vi "OAT Linear Avg Level.vi"(0 "scaled signal [EU]":dbl[](array[numeric]) format="%.2f", 1 "time constant [ms]":dbl=125.0 min=0.0 format="%.2f", 2 "sampling frequency [Hz]":dbl=10000.0 format="%.2f", 4 "init/cont (init:F)":bool) -> (6 "linear avg level [EU^2 rms]":dbl[](array[numeric]) format="%.2f", 7 "actual time constant [ms]":dbl=125.0 format="%.2f")   [LabVIEW 2017, in "SoundVib_Gabor.lvlib"]
doc: "This VI computes the exponential averaged level of the input signal X, based on the selected exponential averaging mode, and returns this level for the entire signal..\n\nThe initial filter state and final filter state keep track of the internal state of the filter to insure continuous operation of the filter (if continuous mode is used)."
uses:
  <vilib>/addons/Sound and Vibration/Order Analysis/Gabor Order Tracking/SoundVib_Gabor.lvlib
  <vilib>/Analysis/3filter.llb/IIR Filter (DBL).vi
  <vilib>/Analysis/NI_AALBase.lvlib
panel:
  in  "exponential mode":enum16{"Slow", "Fast", "Impulse", "Custom"}(ring)=enum."Custom"
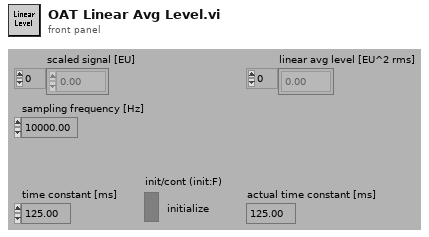
[diagram p1: front panel]
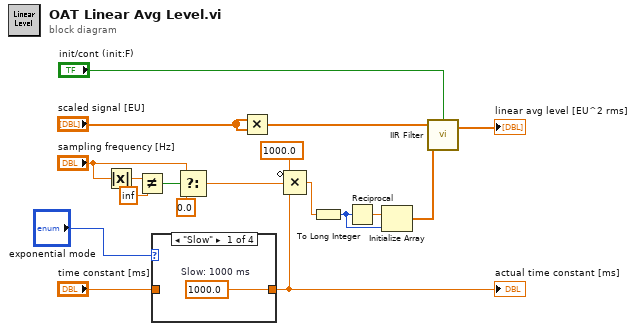
[diagram p0: block diagram]
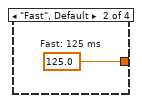
[diagram p2: hidden frame]
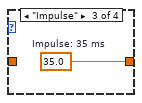
[diagram p3: hidden frame]
diagram:
  n1 = Absolute Value(x="sampling frequency [Hz]") -> (abs(x)=w6:dbl)
  n2 = Not Equal?(x=w6, y=inf) -> (x != y?=w4:bool)
  n3 = case shown="\"Slow\"" "exponential mode" {
    tunnel: [w19 w20 w21 w22] -> w12
    tunnel: "time constant [ms]" -> [_ _ _ w22]
    frame "Slow" {
      w19 = 1000.0  # Slow: 1000 ms
    }
    frame "Fast", Default {
      w20 = 125.0  # Fast: 125 ms
    }
    frame "Impulse" {
      w21 = 35.0  # Impulse: 35 ms
    }
    frame "Custom" {
    }
  }
  "actual time constant [ms]" <- w12
  n4 = Select(t="sampling frequency [Hz]", s=w4, f=0.0) -> (s? t:f=w1:dbl)
  n5 = Multiply(x="scaled signal [EU]", y="scaled signal [EU]") -> (x*y=w9:dbl[])
  n6 = Compound Arithmetic op=MULTIPLY(invert 1000.0 ("Input"), w1, w12) -> (w15:dbl)
  n7 = To Long Integer(number=w15) -> (32bit integer=w13:i32)
  n8 = Reciprocal(x=w13) -> (1/x=w14:dbl)
  n9 = Initialize Array(w14, w13) -> (w10:dbl[])
  n10 = call-poly <vilib>:"IIR Filter.vi"("init/cont (init:F)"="init/cont (init:F)", "Forward Coefficients"=w10, "X"=w9) -> ("Filtered X"=→"linear avg level [EU^2 rms]":dbl[])  [unwired: 1 in, 1 out]
